vi "Stack overflow solution infinite wallet.vi"() -> ()   [LabVIEW 2018]
panel:
  out "Number of solutions":i32 format="%^_6e"
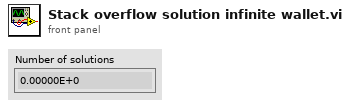
[diagram p1: front panel]
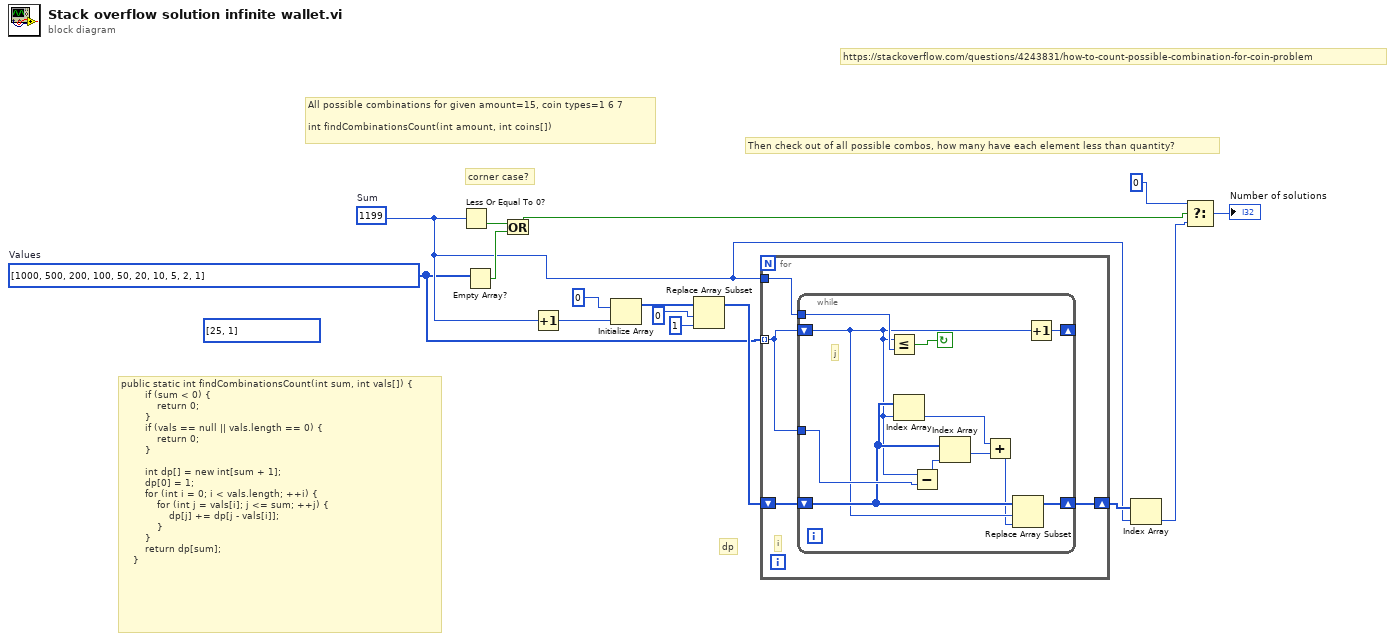
[diagram p0: block diagram]
diagram:
  (unwired) i32[] [25, 1] ("Values")
  w1 = i32[] [1000, 500, 200, 100, 50, 20, 10, 5, 2, 1]  # Values
  w3 = 1199  # Sum
  # "dp"
  # "Then check out of all possible combos, how many have each element less than quantity?"
  # "https://stackoverflow.com/questions/4243831/how-to-count-possible-combination-for-coin-problem"
  # "public static int findCombinationsCount(int sum, int vals[]) {\n        if (sum < 0) {\n            return 0;\n        }\n        if (vals == null || vals.length == 0) {\n            return 0;\n        }\n\n        int dp[] = new int[sum + 1];\n        dp[0] = 1;\n        for (int i = 0; i < vals.length; ++i) {\n            for (int j = vals[i]; j <= sum; ++j) {\n                dp[j] += dp[j - vals[i]];\n            }\n        }\n        return dp[sum];\n    }"
  # "corner case?"
  # "All possible combinations for given amount=15, coin types=1 6 7 \n\nint findCombinationsCount(int amount, int coins[])"
  n1 = Less Or Equal To 0?(x=w3) -> (x <= 0?=w15:bool)
  n2 = Empty Array?(array=w1) -> (empty?=w14:bool)
  n3 = Or(x=w15, y=w14) -> (x .or. y?=w13:bool)
  n4 = Increment(x=w3) -> (x+1=w2:i32)
  n5 = Initialize Array(0 ("element"), w2) -> (w7:i32[])
  n6 = Replace Array Subset(array=w7, new element=1 ("new element/subarray"), index=0) -> (w6:i32[])
  n7 = for {
    tunnel: w1 -> [w17] mode=indexing
    tunnel: w3 -> [w19]
    shift-right: [w16] -> w10
    shift-left: w6 -> [w18]
    # "i"
    n8 = while {
      tunnel: w19 -> [w30]
      shift-right: [w28] -> w16
      shift-left: w18 -> [w24]
      shift-right: [w27] -> _
      shift-left: w17 -> [w23]
      tunnel: w17 -> [w26]
      stop <- w29 continue-if-true
      # "j"
      n9 = Less Or Equal?(x=w23, y=w30) -> (x <= y?=w29:bool)
      n10 = Index Array(array=w24, index=w23) -> (element=w22:i32)
      n11 = Subtract(x=w23, y=w26) -> (x-y=w25:i32)
      n12 = Index Array(array=w24, index=w25) -> (element=w21:i32)
      n13 = Add(x=w22, y=w21) -> (x+y=w20:i32)
      n14 = Replace Array Subset(array=w24, new element=w20, index=w23) -> (w28:i32[])
      n15 = Increment(x=w23) -> (x+1=w27:i32)
    }
  }
  n16 = Index Array(array=w10, index=w3) -> (element=w9:i32)
  n17 = Select(t=0, s=w13, f=w9) -> (s? t:f=→"Number of solutions":i32)
